vi "CalcTorque.vi"(8 "error in (no error)":errorcluster, 11 "CAlexData2 in":refnum<class "CAlexData2.lvclass">) -> (0 "error out":errorcluster, 1 "Joint Torque Actual":dbl[][](array[numeric]), 2 "Joint Torque Desired":dbl[][](array[numeric]), 3 "CAlexData2 out":refnum<class "CAlexData2.lvclass">, 4 "Tension Actual":dbl[][](array[numeric]), 6 "Tension Desired":dbl[][](array[numeric]))   [LabVIEW 2015, in "CAlexData2.lvclass"]
uses:
  CAlexData2.lvclass
  CAlexData2.lvclass/CAlexData2.ctl
  CAlex2/CAlex2.lvclass
  ExpData/ExpData.lvclass
  CableSerialChain/CableSerialChain.lvclass
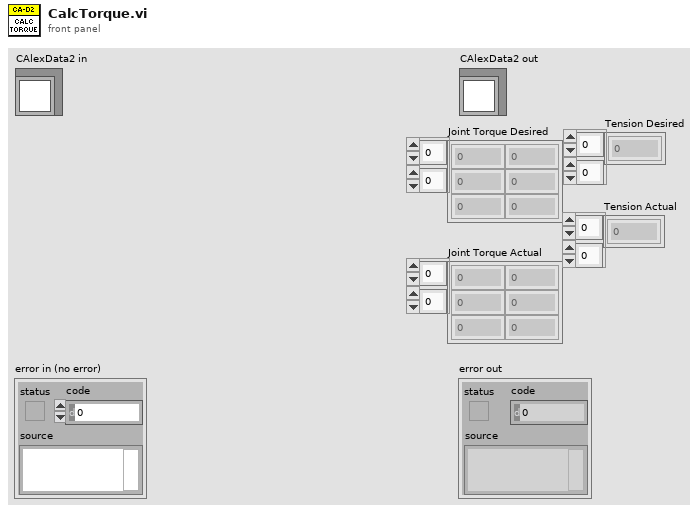
[diagram p1: front panel]
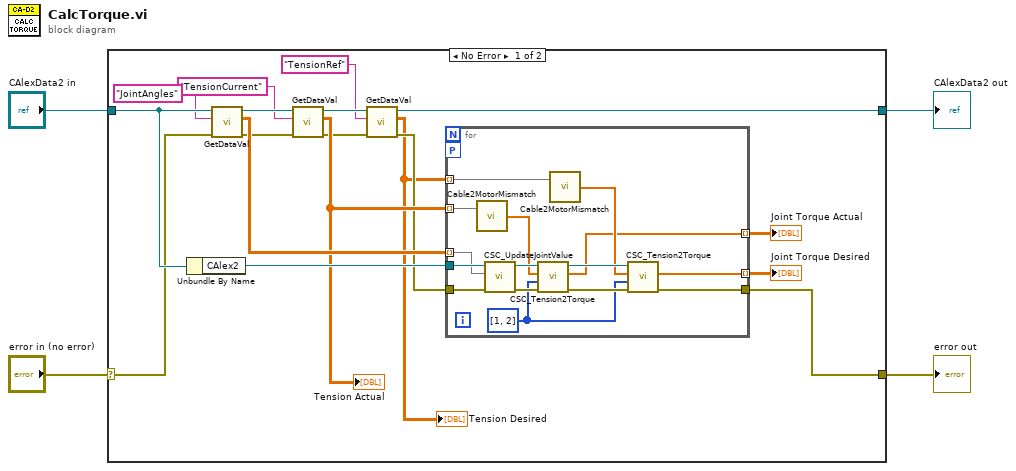
[diagram p0: block diagram]
diagram:
  n1 = case shown="No Error" "error in (no error)" {
    selector: "error in (no error)" -> [w13 w39]
    tunnel: [w12 w39] -> w3
    tunnel: [w9 w38] -> w1
    tunnel: "CAlexData2 in" -> [w21 w38]
    frame No Error {
      n2 = Unbundle By Name(w21) -> ("CAlex2"=w20:refnum<class "CAlex2.lvclass">)
      n3 = call "GetDataVal.vi"("error in (no error)"=w13, "Name"="JointAngles", "CarexMData in"=w21) -> ("error out"=w14:errorcluster, "Data"=w17:dbl[][], "CarexMData out"=w22:refnum<class "CAlexData2.lvclass">)  [unwired: 5 in, 1 out]
      n4 = call "GetDataVal.vi"("error in (no error)"=w14, "Name"="TensionCurrent", "CarexMData in"=w22) -> ("error out"=w8:errorcluster, "Data"=w16:dbl[][], "CarexMData out"=w10:refnum<class "CAlexData2.lvclass">)  [unwired: 5 in, 1 out]
      "Tension Actual" <- w16
      n5 = call "GetDataVal.vi"("error in (no error)"=w8, "Name"="TensionRef", "CarexMData in"=w10) -> ("error out"=w7:errorcluster, "Data"=w6:dbl[][], "CarexMData out"=w9:refnum<class "CAlexData2.lvclass">)  [unwired: 5 in, 1 out]
      "Tension Desired" <- w6
      n6 = for {
        tunnel: w17 -> [w36] mode=indexing
        tunnel: w16 -> [w32] mode=indexing
        tunnel: [w27] -> w15 mode=indexing
        tunnel: w20 -> [w37]
        tunnel: w7 -> [w33]
        tunnel: [w28] -> w12
        workers-P: _ -> [_]
        tunnel: [w25] -> w11 mode=indexing
        tunnel: w6 -> [w24] mode=indexing
        w23 = i32[] [1, 2] ("Locked Joints")
        n7 = call "Cable2MotorMismatch.vi"("MotorTension"=w32) -> ("CableTension"=w31:dbl[])  [unwired: 2 in]
        n8 = call "CSC_UpdateJointValue.vi"("error in (no error)"=w33, "JointValue (rad|m)"=w36, "C-Alex in"=w37) -> ("error out"=w34:errorcluster, "C-Alex out"=w35:refnum<class "CAlex2.lvclass">)  [unwired: 7 in]
        n9 = call-dynamic "CSC_Tension2Torque.vi"("error in (no error)"=w34, "Locked Joints"=w23, "Cable Tensions"=w31, "CSC in"=w35) -> ("error out"=w29:errorcluster, "Joint Torque"=w25:dbl[], "CSC out"=w30:refnum<class "CAlex2.lvclass">)  [unwired: 5 in]
        n10 = call "Cable2MotorMismatch.vi"("MotorTension"=w24) -> ("CableTension"=w26:dbl[])  [unwired: 2 in]
        n11 = call-dynamic "CSC_Tension2Torque.vi"("error in (no error)"=w29, "Locked Joints"=w23, "Cable Tensions"=w26, "CSC in"=w30) -> ("error out"=w28:errorcluster, "Joint Torque"=w27:dbl[])  [unwired: 5 in, 1 out]
      }
      "Joint Torque Desired" <- w15
      "Joint Torque Actual" <- w11
    }
    frame Error {
    }
  }
  "error out" <- w3
  "CAlexData2 out" <- w1
